vi "Inverse Kinematics Demo.vi"() -> ()   [LabVIEW 2017, in "NI_Kinematics.lvlib"]
uses:
  <vilib>/robotics/Kinematics/NI_Kinematics.lvlib
  <vilib>/robotics/Kinematics/Robot/Inverse Kinematics (Trajectory).vi
  <vilib>/robotics/Kinematics/Generate Cartesian Trajectory (Int).vi
panel:
  out "Q":dbl[][](array[numeric])
  out "TR":dbl[][][](array[numeric])
  out "Time (ms)":u32
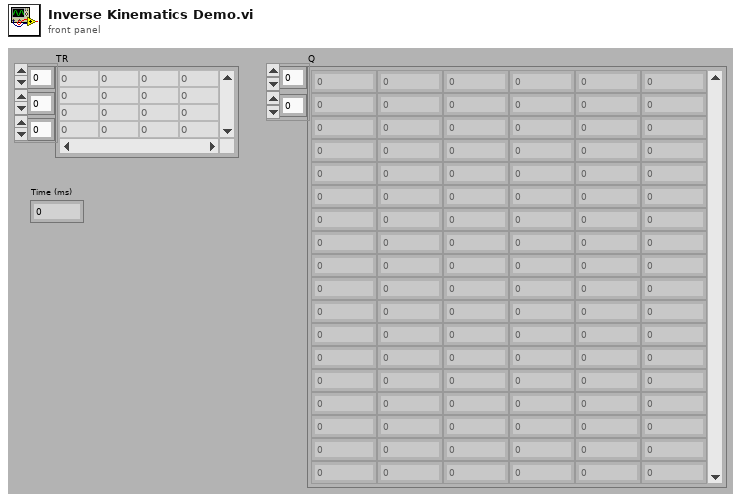
[diagram p1: front panel]
types:
  T1 = typedef "NI_Matrix.lvlib/RealMatrix.ctl" = dbl[][]
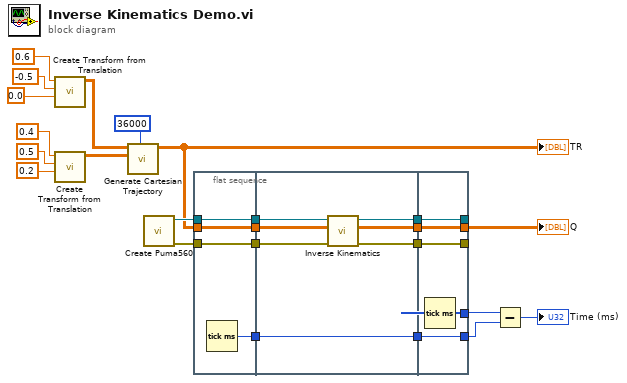
[diagram p0: block diagram]
diagram:
  n1 = call <vilib>:"Create Transform from Translation.vi"("z"=0.0 ("Z"), "y"=-0.5 ("Y"), "x"=0.6 ("X")) -> ("transform"=w5:T1)  [unwired: 1 in, 7 out]
  n2 = call <vilib>:"Create Transform from Translation.vi"("z"=0.2 ("Z"), "y"=0.5 ("Y"), "x"=0.4 ("X")) -> ("transform"=w4:T1)  [unwired: 1 in, 7 out]
  n3 = call-poly <vilib>:"Generate Cartesian Trajectory.vi"("intermediate points"=36000 ("y"), "end transform"=w4, "start transform"=w5) -> ("interpolated trajectory"=w2:dbl[][][])  [unwired: 7 in, 1 out]
  "TR" <- w2
  n4 = call <vilib>:"Create Puma560.vi"() -> ("error out"=w8:errorcluster, "Puma560 Robot"=w18:refnum<class "NI_Robotics_Serial Robot Arm.lvclass">)  [unwired: 1 in, 9 out]
  n5 = flat-sequence {
    tunnel: w2 -> [w27]
    tunnel: w18 -> [w28]
    tunnel: [w28] -> w17
    tunnel: [w27] -> w16
    tunnel: [w26] -> w15
    tunnel: w8 -> [w25]
    tunnel: [w25] -> w7
    tunnel: w17 -> [w30]
    tunnel: w16 -> [w29]
    tunnel: w15 -> [w35]
    tunnel: [w32] -> w14
    tunnel: [w35] -> w13
    tunnel: [w31] -> w9
    tunnel: w7 -> [w34]
    tunnel: [w33] -> w6
    tunnel: [w39] -> w11
    tunnel: [w40] -> w1
    tunnel: w14 -> [w40]
    tunnel: w13 -> [w39]
    tunnel: [w38] -> w12
    tunnel: w9 -> [w37]
    tunnel: [w37] -> _
    tunnel: w6 -> [w36]
    tunnel: [w36] -> _
    frame #0 {
      n6 = Tick Count (ms)() -> (millisecond timer value=w26:u32)
    }
    frame #1 {
      n7 = call-poly <vilib>:"Inverse Kinematics.vi"("error in (no error)"=w34, "end effector trajectory"=w29, "serial arm in"=w30) -> ("error out"=w33:errorcluster, "joint position trajectory"=w32:dbl[][], "serial arm out"=w31:refnum<class "NI_Robotics_Serial Robot Arm.lvclass">)  [unwired: 5 in, 1 out]
    }
    frame #2 {
      n8 = Tick Count (ms)() -> (millisecond timer value=w38:u32)
    }
  }
  n9 = Subtract(x=w12, y=w11) -> (x-y=→"Time (ms)":u32)
  "Q" <- w1
